vi "Save Macro.vi"(8 "error in (no error)":errorcluster, 9 "Macro File (\"File\")":string="File", 10 "Macro Label (\"Label\")":string="Label", 11 "VISA resource name":refnum<visa-resource-name>) -> (0 "error out":errorcluster, 3 "VISA resource name out":refnum<visa-resource-name>)   [LabVIEW 2015, in "Rohde&Schwarz CMXP Base.lvlib"]
doc: "Stores the contents of a macro to a file. If the file exists, it is overwritten. If the file does not exist, it is created.\n\nAttribute:\nRSCMXPBASE_ATTR_SAVE_MACRO\n\nRemote-control command:\nMMEMory:STORe:MACRo"
uses:
  <instrlib>/Rohde&Schwarz CMXP Base/Rohde&Schwarz CMXP Base.lvlib
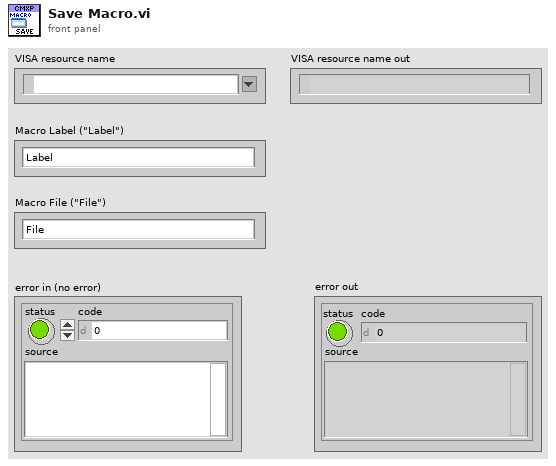
[diagram p1: front panel]
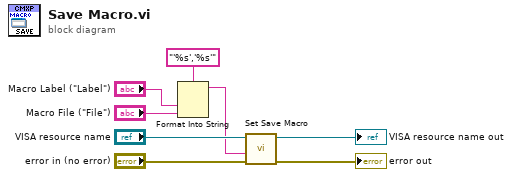
[diagram p0: block diagram]
diagram:
  n1 = Format Into String(format string="'%s','%s'", "Macro Label (\"Label\")", "Macro File (\"File\")") -> (resulting string=w1:string)  [unwired: 2 in, 1 out]
  n2 = call "Set Save Macro"("error in (no error)"="error in (no error)", "Save Macro ()"=w1, "instrument handle"="VISA resource name") -> ("error out"=→"error out":errorcluster, "instrument handle out"=→"VISA resource name out":refnum<visa-resource-name>)  [unwired: 7 in]
